vi "FileWatcher_SPCReader_FDA_v3.vi"(2 "Filenames in":string[](array[string]), 3 "appended path":path) -> (0 "Filesnames out":string[](array[string]), 1 "Raman Spectrum":cluster{i32[], i32[]}(graph))   [LabVIEW 2015]
panel:
  out "Array 2":i32[](array[numeric])
  out "Array":i32[](array[numeric])
  out "new filenames":string[](array[string])
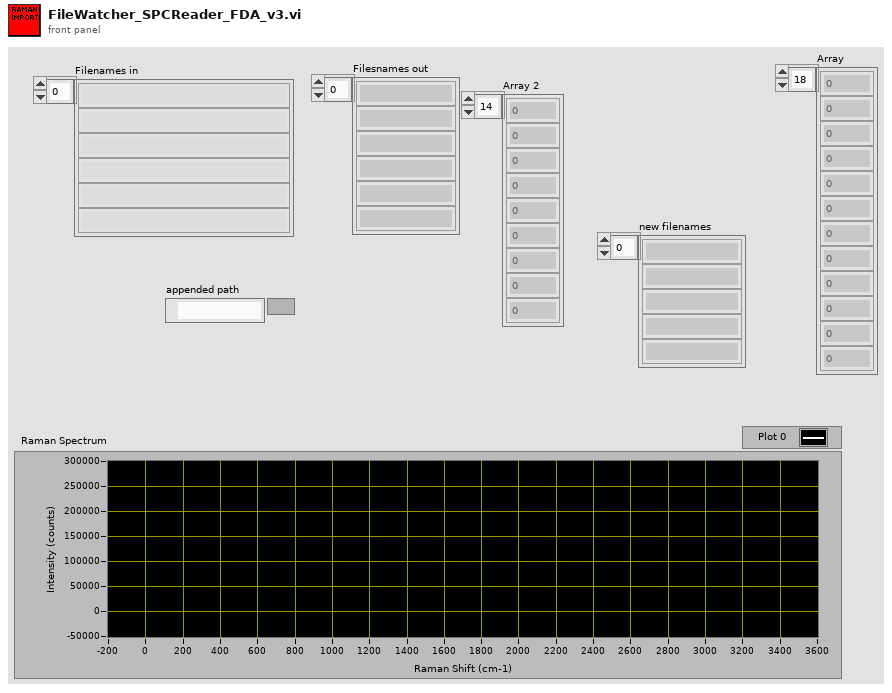
[diagram p1: front panel]
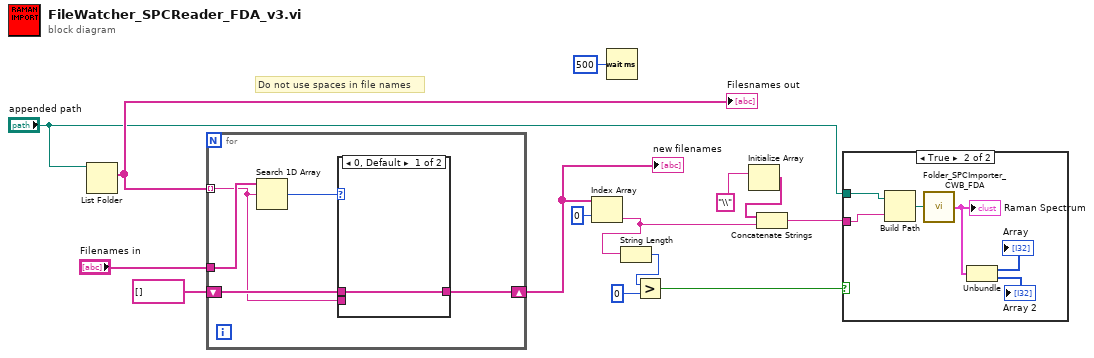
[diagram p0: block diagram]
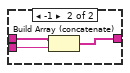
[diagram p2: hidden frame]
diagram:
  # "Do not use spaces in file names"
  n1 = List Folder(path="appended path") -> (filenames=w10:string[])  [unwired: 3 in, 3 out]
  "Filesnames out" <- w10
  n2 = for {
    tunnel: w10 -> [w17] mode=indexing
    tunnel: "Filenames in" -> [w19]
    shift-right: [w15] -> w7
    shift-left: string[] [] ("filenames") -> [w18]
    n3 = Search 1D Array(1D array=w19, element=w17) -> (index of element=w16:i32)  [unwired: 1 in]
    n4 = case shown="0, Default" w16 {
      tunnel: w18 -> [w20 w23]
      tunnel: w17 -> [_ w22]
      tunnel: [w20 w21] -> w15
      frame 0, Default {
      }
      frame -1 {
        n5 = Build Array (concatenate)(w23, w22) -> (w21:string[])
      }
    }
  }
  "new filenames" <- w7
  n6 = Index Array(array=w7, index=0) -> (element=w13:string)
  n7 = Wait (ms)(milliseconds to wait=u32 500) -> ()  [unwired: 1 out]
  n8 = String Length(string=w13) -> (length=w9:i32)
  n9 = Greater?(x=w9, y=0) -> (0:w4:bool)
  n10 = Initialize Array("\\" ("name or relative path")) -> (w12:string[])  [unwired: 1 in]
  n11 = Concatenate Strings(w12, w13) -> (w14:string)
  n12 = case shown="True" w4 {
    tunnel: "appended path" -> [_ w28]
    tunnel: w14 -> [_ w27]
    frame False {
    }
    frame True {
      n13 = Build Path(base path=w28, name or relative path=w27) -> (appended path=w29:path)
      n14 = call "Folder_SPCImporter_CWB_FDA.vi"("Select folder with  .spc files to convert to one .csv file that contains the Raman data and one .csv file that contains to instrument information."=w29) -> ("SPECTRA"=w26:cluster{i32[], i32[]})
      "Raman Spectrum" <- w26
      n15 = Unbundle(w26) -> (→"Array":i32[], →"Array 2":i32[])
    }
  }
